vi "Write UIConfigFileName.vi"(8 "error in (no error)":errorcluster, 10 "UIConfigPath":string, 11 "UI_Top_Customer in":refnum<class "UI_Top_Customer.lvclass">) -> (0 "error out":errorcluster, 3 "UI_Top_Customer out":refnum<class "UI_Top_Customer.lvclass">)   [LabVIEW 2021, in "UI_Top_Customer.lvclass"]
uses:
  UI_Top_Customer.lvclass
  UI_Top_Customer.lvclass/UI_Top_Customer.ctl
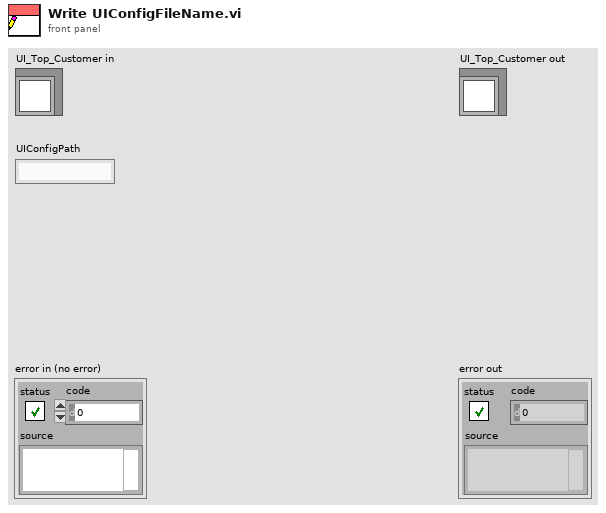
[diagram p1: front panel]
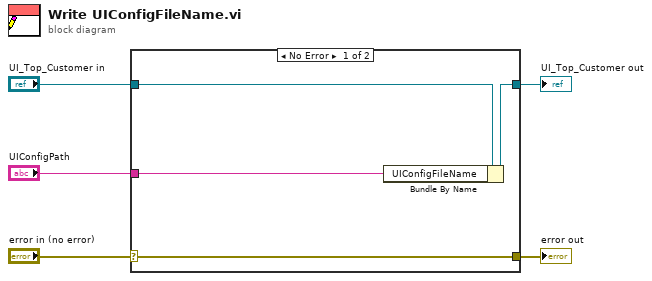
[diagram p0: block diagram]
diagram:
  n1 = case shown="No Error" "error in (no error)" {
    selector: "error in (no error)" -> [w9 w10]
    tunnel: [w9 w10] -> w4
    tunnel: [w7 w11] -> w2
    tunnel: "UI_Top_Customer in" -> [w8 w11]
    tunnel: "UIConfigPath" -> [w6 _]
    frame No Error {
      n2 = Bundle By Name(cluster=w8, "UIConfigFileName"=w6) -> (w7:refnum<class "UI_Top_Customer.lvclass">)
    }
    frame Error {
    }
  }
  "error out" <- w4
  "UI_Top_Customer out" <- w2
